vi "Stop Config.vi"(3 "queue in":refnum<queue>, 5 "SubVI Is Running":i32, 6 "Array":T1[](array[typedef]) {"Private"."Offset" format="%^_3e"; "Private"."Scale Factors" format="%^_3e"}) -> (0 "queue out":refnum<queue>, 2 "Array Out":T1[](array[typedef]) {"Private"."Offset" format="%^_3e"; "Private"."Scale Factors" format="%^_3e"})   [LabVIEW 2019]
uses:
  Sub Controls/Instrument Properties.ctl
  Sub Controls/Public.ctl
  Sub Controls/Private.ctl
  Sub Controls/Instrument Ref.ctl
  Sub Controls/SystemCheckBox-resize.ctl
  Sub Controls/User Event Message.ctl
  Sub Controls/User Event Command.ctl
panel:
  out "Names Out":string[](array[string])
  in  "Names In":string[](array[string])
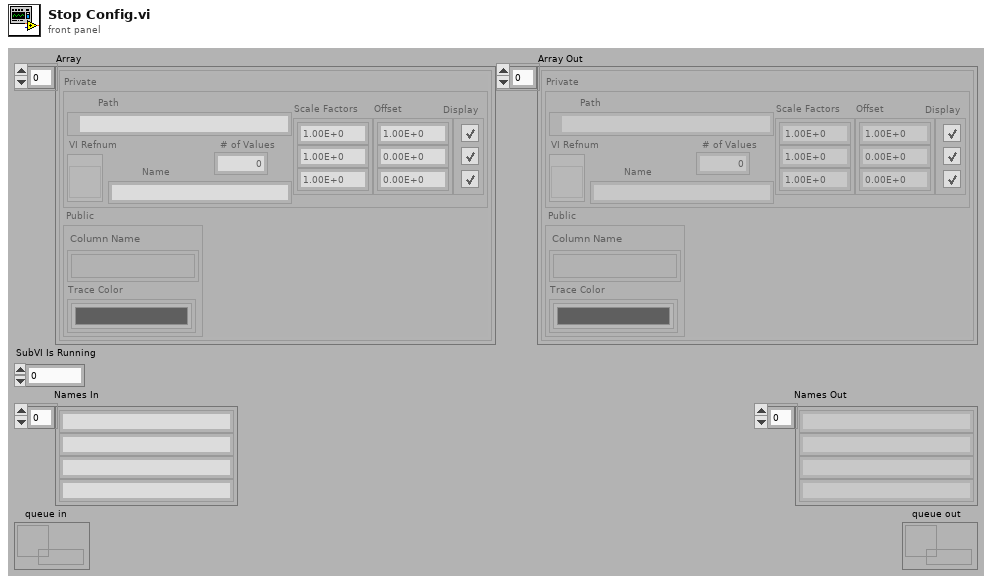
[diagram p1: front panel]
types:
  T1 = typedef "Instrument Properties.ctl" = cluster{"Public":T2, "Private":T3}
  T2 = typedef "Public.ctl" = cluster{"Column Name":string[], "Trace Color":u32[]}
  T3 = typedef "Private.ctl" = cluster{"Path":path, "VI Refnum":T4, "Name":string, "# of Values":i32, "Scale Factors":dbl[], "Display":T5[], "Offset":dbl[]}
  T4 = typedef "Instrument Ref.ctl" = refnum<vi>
  T5 = typedef "SystemCheckBox-resize.ctl" = bool
  T6 = typedef "User Event Message.ctl" = cluster{"Command":T7}
  T7 = typedef "User Event Command.ctl" = enum32{"Stop Config"}
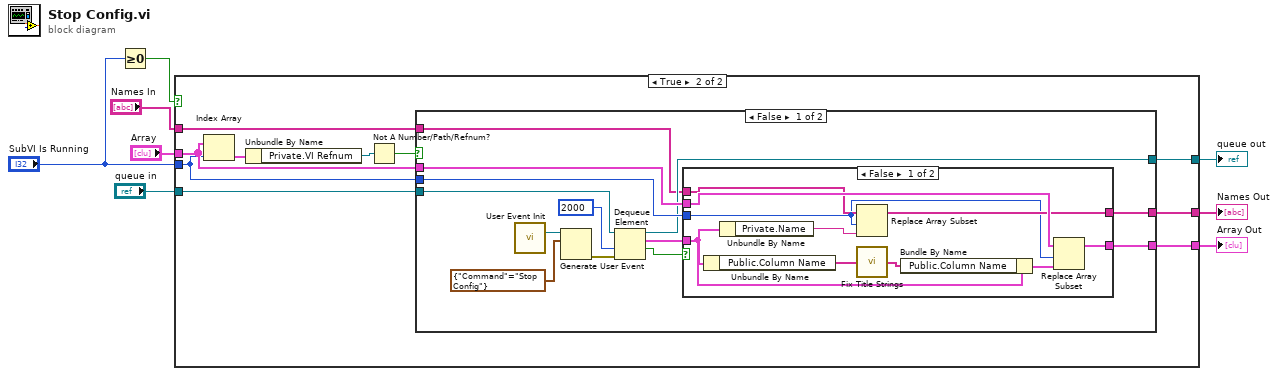
[diagram p0: block diagram]
diagram:
  n1 = Greater Or Equal To 0?(x="SubVI Is Running") -> (x >= 0?=w4:bool)
  n2 = case shown="True" w4 {
    tunnel: [w10 w20] -> w8
    tunnel: "Array" -> [w10 w19]
    tunnel: "queue in" -> [w11 w18]
    tunnel: [w11 w17] -> w5
    tunnel: "SubVI Is Running" -> [_ w14]
    tunnel: [w9 w13] -> w2
    tunnel: "Names In" -> [w9 w12]
    frame False {
    }
    frame True {
      n3 = Index Array(array=w19, index=w14) -> (element=w21:T1)
      n4 = Unbundle By Name(w21) -> ("Private.VI Refnum"=w16:T4)
      n5 = Not A Number/Path/Refnum?(number/path/refnum=w16) -> (NaN/Path/Refnum?=w15:bool)
      n6 = case shown="False" w15 {
        tunnel: [w34 w49] -> w20
        tunnel: w19 -> [w33 w49]
        tunnel: w14 -> [w32 _]
        tunnel: w18 -> [w31 w48]
        tunnel: [w30 w48] -> w17
        tunnel: [w23 w47] -> w13
        tunnel: w12 -> [w22 w47]
        frame False {
          n7 = call "User Event Init.vi"() -> ("main menu User Event"=w29:refnum<user-event>)  [unwired: 14 in, 1 out]
          n8 = Generate User Event(user event=w29, event data cluster=T6 {"Command"=enum."Stop Config"} ("event data")) -> (error out=w26:errorcluster)  [unwired: 2 in, 1 out]
          n9 = Dequeue Element(queue=w31, timeout in ms (-1)=2000, error in (no error)=w26) -> (queue out=w30:refnum<queue>, element=w27:T1, timed out?=w24:bool)  [unwired: 1 out]
          n10 = case shown="False" w24 {
            tunnel: [w44 w46] -> w34
            tunnel: w33 -> [w43 w46]
            tunnel: w32 -> [w40 _]
            tunnel: w27 -> [w38 _]
            tunnel: [w42 w45] -> w23
            tunnel: w22 -> [w41 w45]
            frame False {
              n11 = Unbundle By Name(w38) -> ("Public.Column Name"=w36:string[])
              n12 = Unbundle By Name(w38) -> ("Private.Name"=w39:string)
              n13 = Replace Array Subset(array=w41, new element=w39, index=w40) -> (w42:string[])
              n14 = call "Fix Title Strings.vi"("Title In"=w36) -> ("Title Out"=w35:string[])
              n15 = Bundle By Name(cluster=w38, "Public.Column Name"=w35) -> (w37:T1)
              n16 = Replace Array Subset(array=w43, new element=w37, index=w40) -> (w44:T1[])
            }
            frame True {
            }
          }
        }
        frame True {
        }
      }
    }
  }
  "Array Out" <- w8
  "queue out" <- w5
  "Names Out" <- w2
